vi "STOP_WATCH.vi"(0 "Variable":i32, 5 "Switch":bool, 7 "RESET":bool) -> (4 "Time (Sec)":i32)   [LabVIEW 2025]
doc: "This VI adds 1 for every second LED is ON"
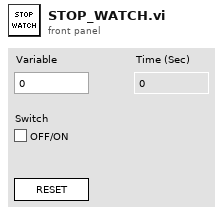
[diagram p1: front panel]
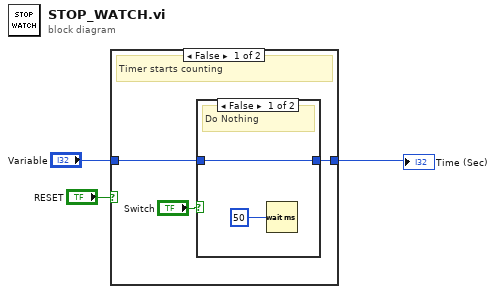
[diagram p0: block diagram]
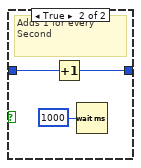
[diagram p2: hidden frame]
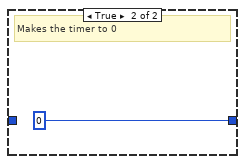
[diagram p3: hidden frame]
diagram:
  n1 = case shown="False" "RESET" {
    tunnel: "Variable" -> [w5 _]
    tunnel: [w4 0] -> w1
    frame False {
      # "Timer starts counting"
      n2 = case shown="False" "Switch" {
        tunnel: w5 -> [w8 w11]
        tunnel: [w8 w9] -> w4
        frame False {
          # "Do Nothing"
          n3 = Wait (ms)(milliseconds to wait=u32 50) -> ()  [unwired: 1 out]
        }
        frame True {
          # "Adds 1 for every Second"
          n4 = Increment(x=w11) -> (x+1=w9:i32)
          n5 = Wait (ms)(milliseconds to wait=u32 1000) -> ()  [unwired: 1 out]
        }
      }
    }
    frame True {
      # "Makes the timer to 0"
    }
  }
  "Time (Sec)" <- w1
